vi "Verbosity - dialog gate.vi"(8 "error in (no error)":errorcluster) -> (0 "error out":errorcluster)   [LabVIEW 2026, in "Tests.lvlib"]
doc: "Unit test (Caraya): verifies ShouldDisplay maps (errorSeverity, verbosity) to the General Error Handler dialog-type selector, so the verbosity gate is proven correct without rendering a modal (SRS-LMBR-042).\nDrives ShouldDisplay across a severity x verbosity grid and asserts dialogType: shown (1) when the error is at least as severe as the verbosity threshold, i.e. rank(errorSeverity) <= rank(verbosity); suppressed (0) otherwise. Covers the inclusive boundary (error = verbosity), one above, one below, and the OFF and ALL extremes.\nTests.lvlib, friend of Lumberjack.lvlib; unit tier, runs in parallel with errors merged.\n\nImplements LMBR-T-055 -> SRS-042. Assert-level IDs: Test-ID-Assert-Checklist.md."
uses:
  Tests.lvlib
  src/TypeDefs/Severity.ctl
  <vilib>/addons/_JKI Toolkits/Caraya/classes/Assert/Assert True.vi
  <vilib>/addons/_JKI Toolkits/Caraya/classes/Assert/Assert False.vi
  src/Lumberjack.lvlib
  <vilib>/addons/_JKI Toolkits/Caraya/classes/Assert/Assert.lvclass
  <vilib>/addons/_JKI Toolkits/Caraya/classes/Test/Test.lvclass
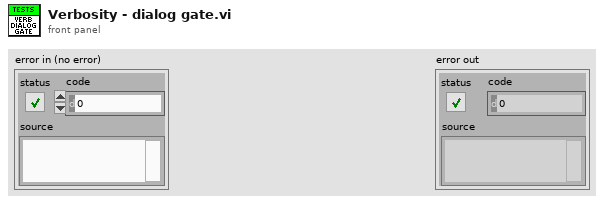
[diagram p1: front panel]
types:
  T1 = typedef "Lumberjack.lvlib/Severity.ctl" = enum16{"OFF", "FATAL", "ERROR", "WARN", "INFO", "DEBUG", "TRACE", "ALL"}
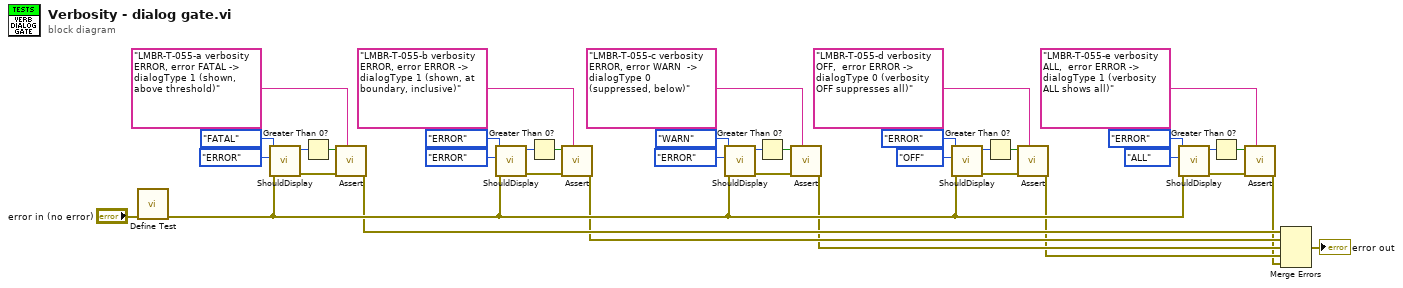
[diagram p0: block diagram]
diagram:
  n1 = call <vilib>:"Define Test.vi"("error in (no error)"="error in (no error)") -> ("error out"=w18:errorcluster)  [unwired: 9 in, 1 out]
  n2 = call "ShouldDisplay.vi"("error in (no error)"=w18, "verbosity"=Severity."ERROR" ("Level"), "errorSeverity"=Severity."FATAL" ("Level")) -> ("error out"=w36:errorcluster, "dialogType"=w10:i32)  [unwired: 7 in]
  n3 = Greater Than 0?(x=w10) -> (x > 0?=w9:bool)
  n4 = call-poly <vilib>:"Assert.vi"("Label"="LMBR-T-055-a verbosity ERROR, error FATAL -> dialogType 1 (shown, above threshold)", "error in (no error)"=w36, "True?"=w9) -> ("error out"=w17:errorcluster)  [unwired: 7 in, 1 out]
  n5 = call "ShouldDisplay.vi"("error in (no error)"=w18, "verbosity"=Severity."ERROR" ("Level"), "errorSeverity"=Severity."ERROR" ("Level")) -> ("error out"=w32:errorcluster, "dialogType"=w8:i32)  [unwired: 7 in]
  n6 = Greater Than 0?(x=w8) -> (x > 0?=w7:bool)
  n7 = call-poly <vilib>:"Assert.vi"("Label"="LMBR-T-055-b verbosity ERROR, error ERROR -> dialogType 1 (shown, at boundary, inclusive)", "error in (no error)"=w32, "True?"=w7) -> ("error out"=w16:errorcluster)  [unwired: 7 in, 1 out]
  n8 = call "ShouldDisplay.vi"("error in (no error)"=w18, "verbosity"=Severity."ERROR" ("Level"), "errorSeverity"=Severity."WARN" ("Level")) -> ("error out"=w28:errorcluster, "dialogType"=w6:i32)  [unwired: 7 in]
  n9 = Greater Than 0?(x=w6) -> (x > 0?=w5:bool)
  n10 = call-poly <vilib>:"Assert.vi"("Label"="LMBR-T-055-c verbosity ERROR, error WARN  -> dialogType 0 (suppressed, below)", "error in (no error)"=w28, "False?"=w5) -> ("error out"=w15:errorcluster)  [unwired: 7 in, 1 out]
  n11 = call "ShouldDisplay.vi"("error in (no error)"=w18, "verbosity"=Severity."OFF" ("Level"), "errorSeverity"=Severity."ERROR" ("Level")) -> ("error out"=w24:errorcluster, "dialogType"=w4:i32)  [unwired: 7 in]
  n12 = Greater Than 0?(x=w4) -> (x > 0?=w3:bool)
  n13 = call-poly <vilib>:"Assert.vi"("Label"="LMBR-T-055-d verbosity OFF,  error ERROR -> dialogType 0 (verbosity OFF suppresses all)", "error in (no error)"=w24, "False?"=w3) -> ("error out"=w14:errorcluster)  [unwired: 7 in, 1 out]
  n14 = call "ShouldDisplay.vi"("error in (no error)"=w18, "verbosity"=Severity."ALL" ("Level"), "errorSeverity"=Severity."ERROR" ("Level")) -> ("error out"=w20:errorcluster, "dialogType"=w2:i32)  [unwired: 7 in]
  n15 = Greater Than 0?(x=w2) -> (x > 0?=w1:bool)
  n16 = call-poly <vilib>:"Assert.vi"("Label"="LMBR-T-055-e verbosity ALL,  error ERROR -> dialogType 1 (verbosity ALL shows all)", "error in (no error)"=w20, "True?"=w1) -> ("error out"=w13:errorcluster)  [unwired: 7 in, 1 out]
  n17 = Merge Errors(w17, w16, w15, w14, w13) -> (→"error out":errorcluster)
